vi "Pit Scouting.vi"() -> ()   [LabVIEW 2016]
uses:
  <vilib>/Utility/sysdir.llb/System Directory Type.ctl
panel:
  in  "?":bool
  in  "Fuel per eighth of second":dbl
  in  "What is your strategy?":string
  in  "Top or bottom goal?":string(combo)
  in  "Can it fuel?":bool
  in  "What kind of power?":string
  in  "How many wheels?":dbl
  in  "What is your robot capable of doing during a match?":string
  in  "How many drive trains?":dbl
  in  "What kind of drive train?":string
  in  "Autonomous?":bool
  in  "Picks up gears?":bool
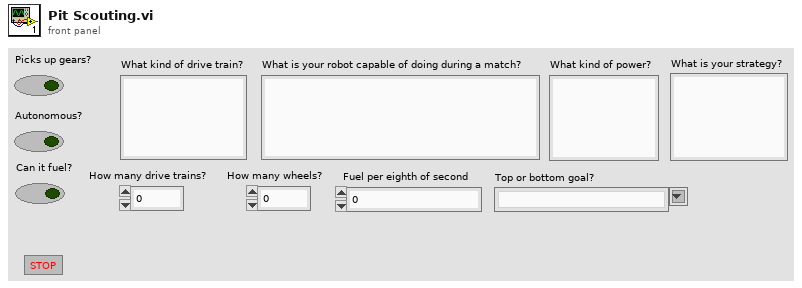
[diagram p1: front panel]
types:
  T1 = typedef "System Directory Type.ctl" = i32
  T2 = enum16{"open", "replace", "create", "open or create", "replace or create", "replace or create with confirmation"}
  T3 = enum32{"invalid app kind", "Development System", "Run Time System", "Student Edition", "Embedded LabVIEW", "Evaluation", "Custom"}
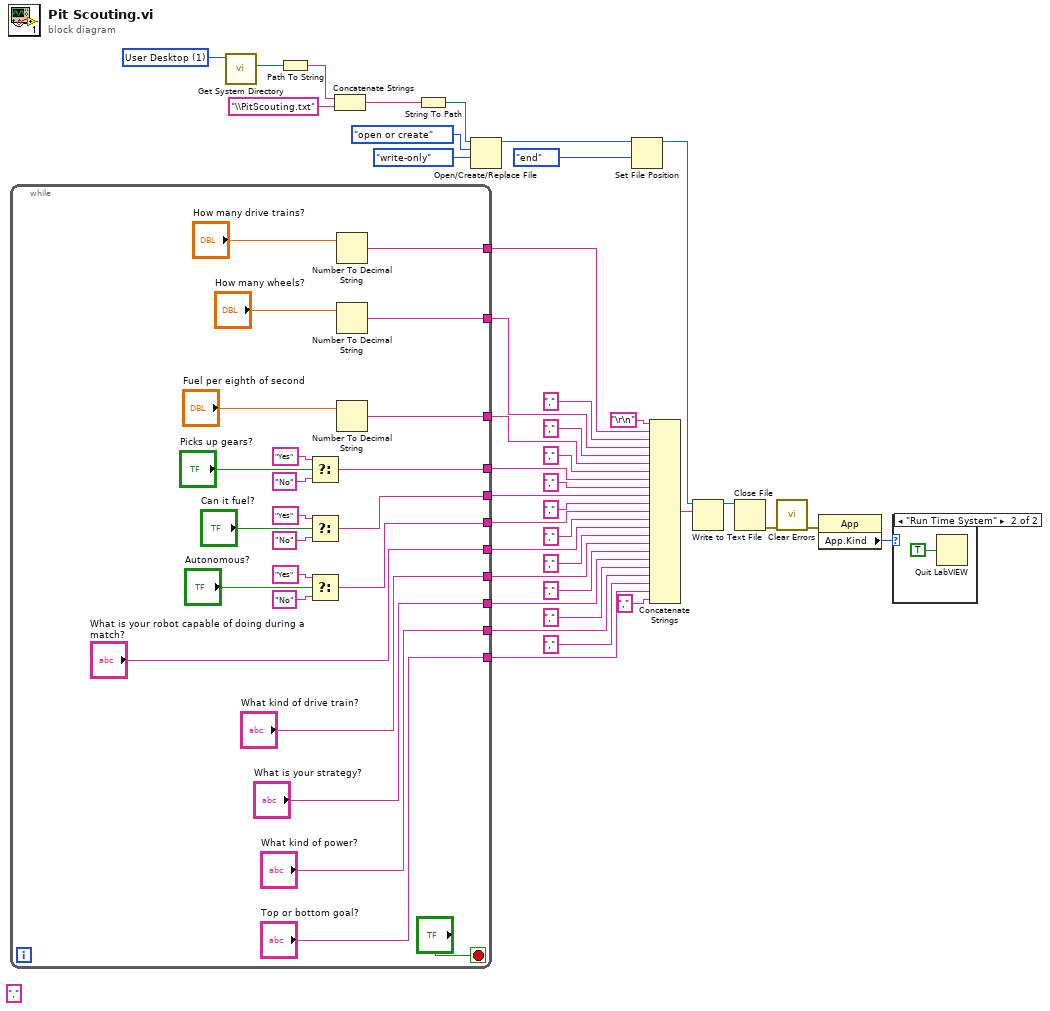
[diagram p0: block diagram]
diagram:
  w35 = T1 1 items=["User Home"=0, "User Desktop"=1, "User Documents"=2, "User Application Data"=3, "User Preferences"=4, "User Temporary"=5, "Public Documents"=6, "Public Application Data"=7, "Public Preferences"=8, "Public Cache"=13, "System Core Libraries"=9, "System Installed Libraries"=10, "Application Files"=11, "Boot Volume Root"=12] ("system directory type")
  (unwired) ","
  n1 = while {
    tunnel: [w53] -> w22
    tunnel: [w52] -> w20
    tunnel: [w51] -> w18
    tunnel: [w50] -> w16
    tunnel: [w49] -> w14
    tunnel: [w48] -> w12
    tunnel: ["What is your robot capable of doing during a match?"] -> w10
    tunnel: ["What kind of drive train?"] -> w9
    tunnel: ["What is your strategy?"] -> w6
    tunnel: ["What kind of power?"] -> w4
    tunnel: ["Top or bottom goal?"] -> w2
    stop <- "?" stop-if-true
    n2 = Select(t="Yes", s="Picks up gears?", f="No") -> (s? t:f=w50:string)
    n3 = Select(t="Yes", s="Can it fuel?", f="No") -> (s? t:f=w49:string)
    n4 = Select(t="Yes", s="Autonomous?", f="No") -> (s? t:f=w48:string)
    n5 = Number To Decimal String(number="How many drive trains?") -> (decimal integer string=w53:string)  [unwired: 1 in]
    n6 = Number To Decimal String(number="How many wheels?") -> (decimal integer string=w52:string)  [unwired: 1 in]
    n7 = Number To Decimal String(number="Fuel per eighth of second") -> (decimal integer string=w51:string)  [unwired: 1 in]
  }
  n8 = call <vilib>:"Get System Directory.vi"("system directory type"=w35) -> ("system directory"=w34:path)  [unwired: 10 in]
  n9 = Path To String(path=w34) -> (string=w33:string)
  n10 = Concatenate Strings(w33, "\\PitScouting.txt" ("string")) -> (w31:string)
  n11 = String To Path(string=w31) -> (path=w30:path)
  n12 = Open/Create/Replace File(file path (use dialog)=w30, operation (0:open)=T2."open or create", access (0:read/write)=enum16{"read/write", "read-only", "write-only"}."write-only") -> (refnum out=w37:refnum<file>)  [unwired: 3 in, 2 out]
  n13 = Set File Position(refnum=w37, from (0:start)=enum16{"start", "end", "current"}."end") -> (refnum out=w25:refnum<file>)  [unwired: 2 in, 1 out]
  n14 = Concatenate Strings("\r\n", w22, ",", w20, ",", w18, ",", w16, ",", w14, ",", w12, ",", w10, ",", w9, ",", w6, ",", w4, ",", w2, ",") -> (w24:string)
  n15 = Write to Text File(file (use dialog)=w25, text=w24) -> (refnum out=w29:refnum<file>)  [unwired: 2 in, 2 out]
  n16 = Close File(refnum=w29) -> (error out=w28:errorcluster)  [unwired: 1 in, 1 out]
  n17 = call <vilib>:"Clear Errors.vi"("error in (no error)"=w28) -> ("error out"=w27:errorcluster)  [unwired: 5 in, 1 out]
  n18 = property class="App"(error in=w27) -> ("App.Kind"=w26:T3)  [unwired: 1 in, 2 out]
  n19 = case shown="\"Run Time System\"" w26 {
    frame Default {
    }
    frame "Run Time System" {
      n20 = Quit LabVIEW(quit? (T)=TRUE) -> ()
    }
  }
